vi "N4_201.vi"(4 "error in":T15, 7 "Command":T16) -> (0 "error out":T15, 3 "Response":T13)   [LabVIEW 2018]
uses:
  MOKO_LabViewLibrary/MokoLowLevel/MokoLowLovelControl/MLLC_Command.ctl
  MOKO_LabViewLibrary/MokoLowLevel/MokoLowLovelControl/MLLC_Error.ctl
  MOKO_LabViewLibrary/MokoLowLevel/MokoLowLovelControl/MLLC_Mode.ctl
  MOKO_LabViewLibrary/MokoLowLevel/MokoLowLovelControl/MLLC_Response.ctl
  MOKO_LabViewLibrary/MokoLowLevel/MokoLowLovelControl/MLLC_DriverName.ctl
  MOKO_LabViewLibrary/MokoLowLevel/MokoLowLovelControl/MLLC_Request.ctl
  MOKO_LabViewLibrary/MokoLowLevel/MokoLowLovelControl/MLLC_ErrorCode.ctl
  MOKO_LabViewLibrary/MokoLowLevel/MokoLowLovelControl/MLLC_ResponseInit.ctl
  MOKO_LabViewLibrary/MokoLowLevel/MokoLowLovelControl/MLLC_ConnectCluster.ctl
  MOKO_LabViewLibrary/MokoLowLevel/MokoLowLovelControl/MLLC_InterfaceType.ctl
  MOKO_LabViewLibrary/MokoLowLevel/MokoLowLovelControl/MLLC_OpenedSession.ctl
  MOKO_LabViewLibrary/MokoLowLevel/MokoLowLovelControl/MLLC_InterfaceSettings.ctl
  MOKO_LabViewLibrary/MokoLowLevel/MokoLowLovelControl/MLLC_InterfaceKind.ctl
  MOKO_LabViewLibrary/MokoLowLevel/MokoLowLovelControl/MLLC_Boolean.ctl
  MOKO_LabViewLibrary/MokoLowLevel/MokoLowLovelControl/MLLC_Delay.ctl
panel:
  in  "Settings":T8={"Connect"={"InterfaceType"=enum."VISA", "OpenedSession"="COM1", "InterfaceSettings"={"Interface"=enum."RS232", "EOS 4 read"=enum."LF (\\n)", "EOS 4 write"=enum."LF (\\n)", "TMO, ms"=10000, "Sett"=variant(cluster{"Baud Rate":u32, "Data Bits":u16, "Parity":u16, "Stop Bits":u16, "Flow Control":u16, "Eho":bool} {"Baud Rate"=75, "Data Bits"=0, "Parity"=0, "Stop Bits"=0, "Flow Control"=0, "Eho"=FALSE})}}, "SwitchOFF"=TRUE, "RangeAuto"=TRUE, "Range"=0.0}
  in  "ResponseInit":T9="N4-201"
  in  "Error Code":T10=5470
  in  "Request":T11="IDN?\n"
  in  "Driver Name":T12="N4_201"
  in  "Mode":T14=enum."Check"
  # "N4-201"
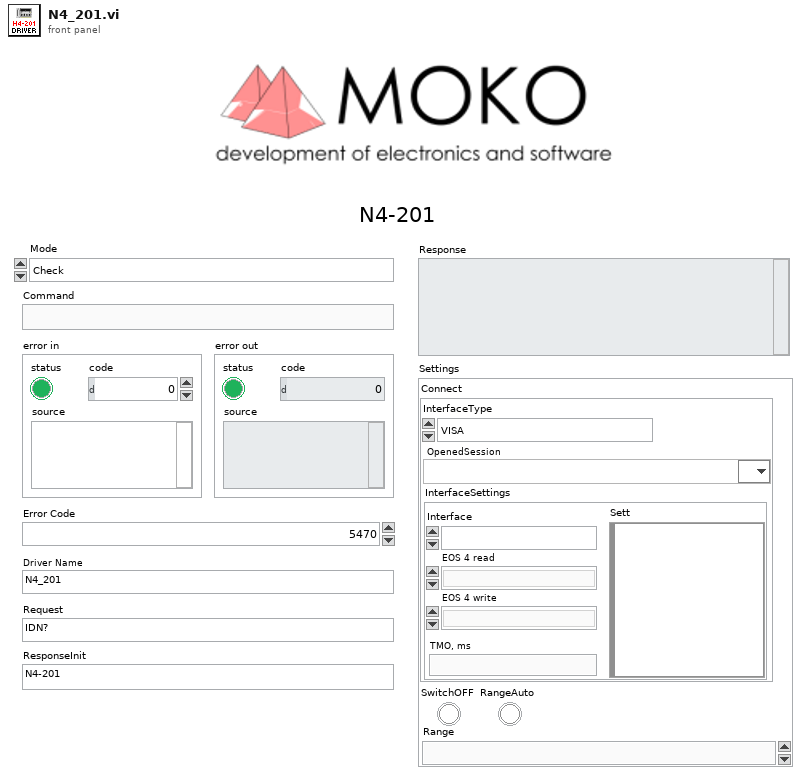
[diagram p1: front panel]
types:
  T1 = typedef "MLLC_ConnectCluster.ctl" = cluster{"InterfaceType":T2, "OpenedSession":T3, "InterfaceSettings":T4}
  T2 = typedef "MLLC_InterfaceType.ctl" = enum16{"VISA", "Prologix USB-GPIB"}
  T3 = typedef "MLLC_OpenedSession.ctl" = refnum<visa-resource-name>
  T4 = typedef "MLLC_InterfaceSettings.ctl" = cluster{"Interface":T5, "EOS 4 read":enum16{"Default (=EOS 4 write)", "CR (\\r)", "LF (\\n)", "None"}, "EOS 4 write":enum16{"CR+LF (\\r\\n)", "CR (\\r)", "LF (\\n)", "None"}, "TMO, ms":i32, "Sett":variant}
  T5 = typedef "MLLC_InterfaceKind.ctl" = enum16{"RS232", "GPIB", "USB", "Ethernet", "another"}
  T6 = typedef "MLLC_Boolean.ctl" = bool
  T7 = typedef "MLLC_Delay.ctl" = dbl
  T8 = cluster{"Connect":T1, "SwitchOFF":T6, "RangeAuto":T6, "Range":T7}
  T9 = typedef "MLLC_ResponseInit.ctl" = string
  T10 = typedef "MLLC_ErrorCode.ctl" = u32
  T11 = typedef "MLLC_Request.ctl" = string
  T12 = typedef "MLLC_DriverName.ctl" = string
  T13 = typedef "MLLC_Response.ctl" = string
  T14 = typedef "MLLC_Mode.ctl" = enum16{"get", "set", "close", "Init", "Check"}
  T15 = typedef "MLLC_Error.ctl" = errorcluster
  T16 = typedef "MLLC_Command.ctl" = string
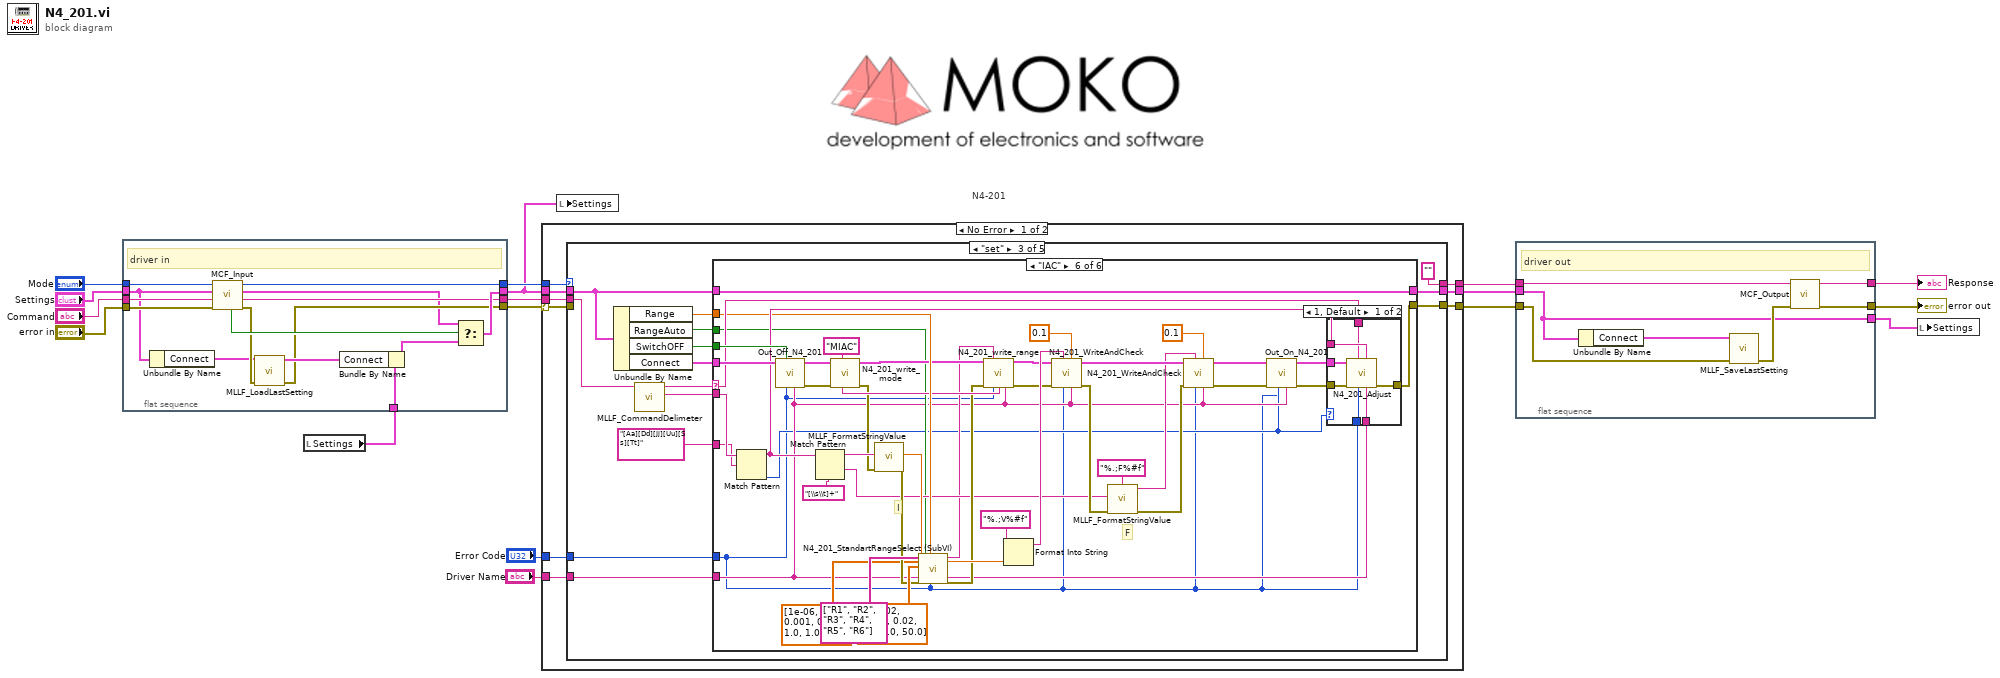
[diagram p0: block diagram]
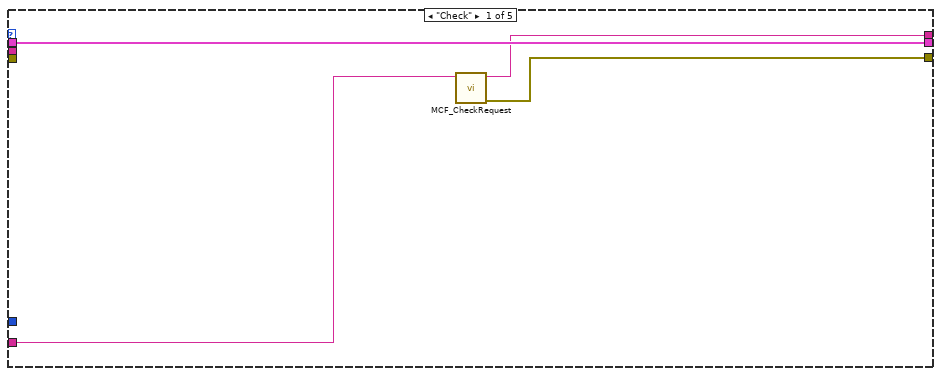
[diagram p2: hidden frame]
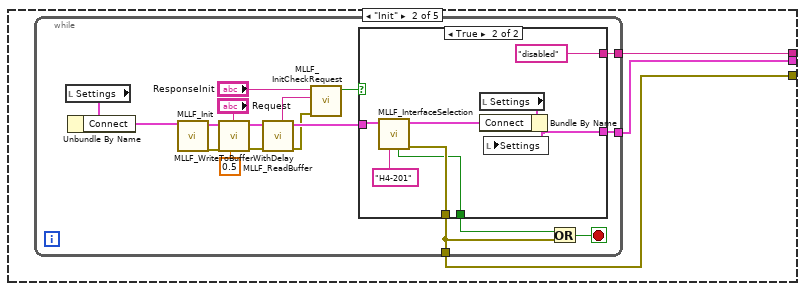
[diagram p3: hidden frame]
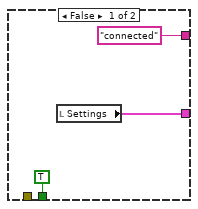
[diagram p4: hidden frame]
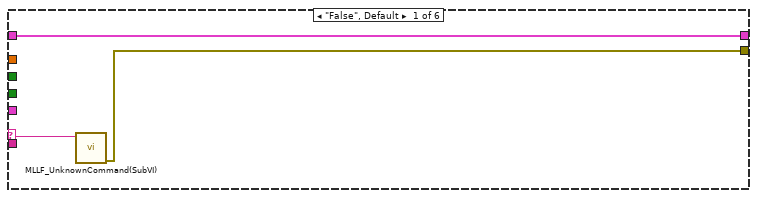
[diagram p5: hidden frame]
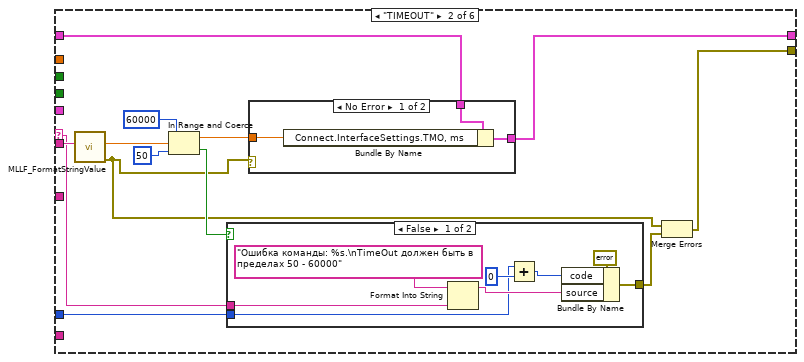
[diagram p6: hidden frame]
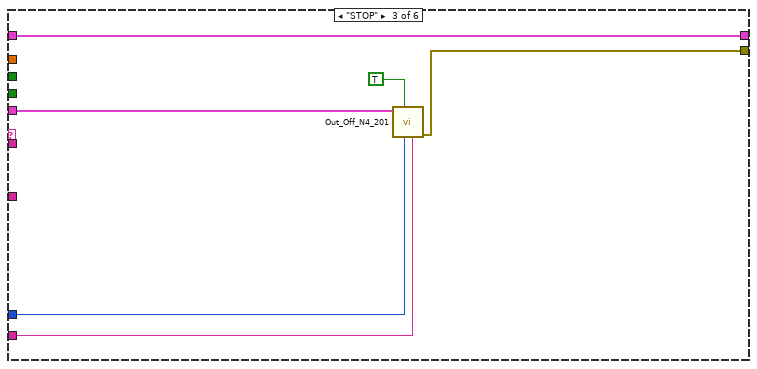
[diagram p9: hidden frame]
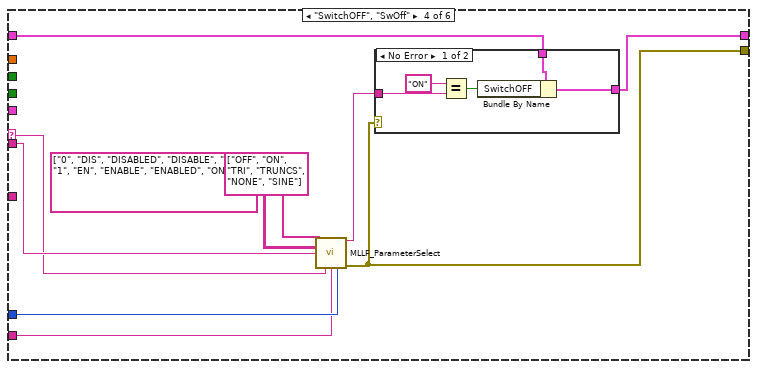
[diagram p10: hidden frame]
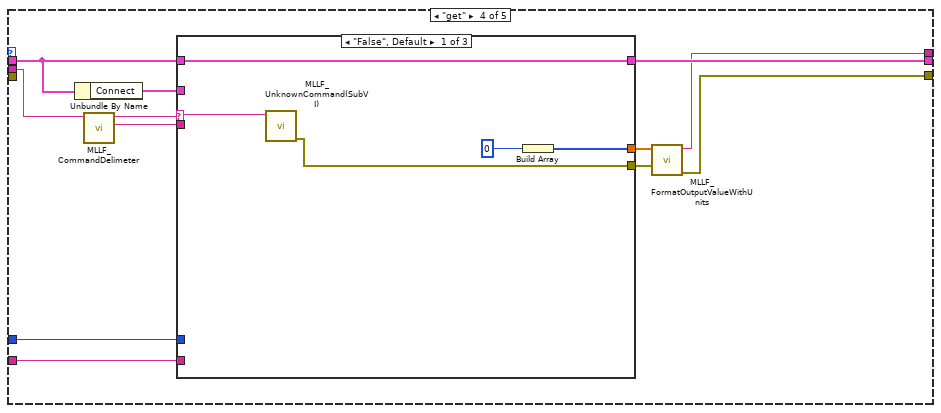
[diagram p14: hidden frame]
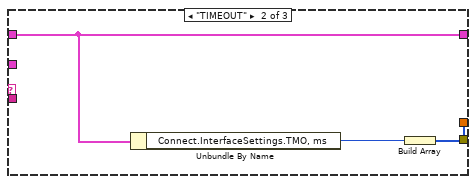
[diagram p15: hidden frame]
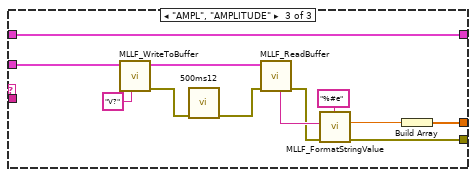
[diagram p16: hidden frame]
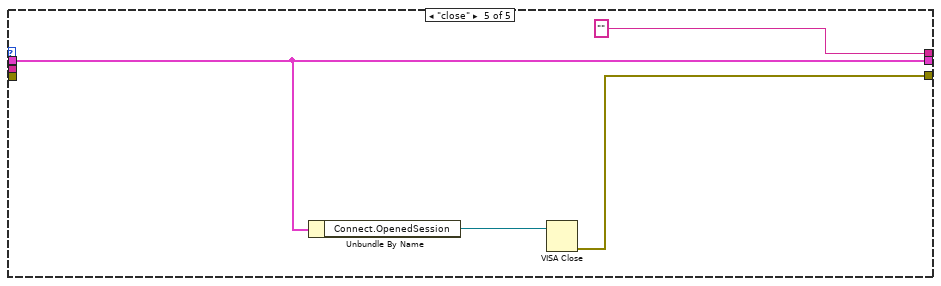
[diagram p17: hidden frame]
diagram:
  # "N4-201"
  n1 = flat-sequence {
    tunnel: [w24] -> w10
    tunnel: "Command" -> [w25]
    tunnel: "Mode" -> [w27]
    tunnel: "Settings" -> [w19]
    tunnel: [w29] -> w2
    tunnel: w1 -> [w28]
    tunnel: "error in" -> [w22]
    tunnel: [w21] -> w15
    tunnel: [w20] -> w9
    frame #0 {
      # "driver in"
      n2 = Unbundle By Name(w19) -> ("Connect"=w18:T1)
      n3 = call "MCF_Input.vi"("error in (no error)"=w22, "Command"=w25, "Mode"=w27) -> ("error out"=w23:errorcluster, "Command out"=w24:string, "Mode out"=w21:T14, "Boolean"=w26:bool)  [unwired: 5 in]
      n4 = call "MLLF_LoadLastSetting.vi"("Error In"=w23, "DriverConnectCluster in"=w18) -> ("Error Out"=w20:errorcluster, "DriverConnectCluster out"=w30:T1)  [unwired: 8 in]
      n5 = Bundle By Name(cluster=w28, "Connect"=w30) -> (w31:T8)
      n6 = Select(t=w19, s=w26, f=w31) -> (s? t:f=w29:T8)
    }
  }
  n7 = local read "Settings"() -> (w1:T8)
  n8 = case shown="No Error" w9 {
    selector: w9 -> [w36 w231]
    tunnel: [w38 w231] -> w6
    tunnel: w15 -> [w40 _]
    tunnel: [w39 _] -> w8
    tunnel: w10 -> [w37 _]
    tunnel: w2 -> [w33 w230]
    tunnel: "Error Code" -> [w35 _]
    tunnel: "Driver Name" -> [w34 _]
    tunnel: [w32 w230] -> w7
    frame No Error {
      n9 = case shown="\"set\"" w40 {
        tunnel: [w42 w47 "" ("String") w195 "" ("String")] -> w39
        tunnel: [w43 w45 w77 w194 w228] -> w38
        tunnel: w37 -> [_ _ w90 w205 _]
        tunnel: w36 -> [_ _ _ _ _]
        tunnel: w35 -> [_ _ w89 w202 _]
        tunnel: w34 -> [w41 _ w86 w201 _]
        tunnel: w33 -> [w44 _ w88 w204 w227]
        tunnel: [w44 w46 w87 w203 w227] -> w32
        frame "Check" {
          n10 = call "MCF_CheckRequest.vi"("Driver Name"=w41) -> ("Error Out"=w43:errorcluster, "Output String"=w42:string)  [unwired: 9 in]
        }
        frame "Init" {
          n11 = while {
            tunnel: [w58] -> w45
            tunnel: [w49] -> w46
            tunnel: [w48] -> w47
            stop <- w56 stop-if-true
            n12 = local read "Settings"() -> (w65:T8)
            n13 = Unbundle By Name(w65) -> ("Connect"=w59:T1)
            n14 = call "MLLF_Init.vi"("DriverConnect in"=w59) -> ("Error Out"=w61:errorcluster, "DriverConnect out"=w60:T1)  [unwired: 7 in]
            n15 = call "MLLF_WriteToBufferWithDelay.vi"("Delay Time ( 0,05 s)"=0.5 ("Delay Time (s)"), "Command"="Request", "Error In"=w61, "DriverConnect in"=w60) -> ("Error Out"=w54:errorcluster, "DriverConnect out"=w63:T1)  [unwired: 6 in]
            n16 = call "MLLF_ReadBuffer.vi"("Error In"=w54, "DriverConnect in"=w63) -> ("Error Out"=w51:errorcluster, "DriverConnect out"=w62:T1, "String"=w52:string)  [unwired: 6 in]
            n17 = call "MLLF_InitCheckRequest.vi"("error in (no error)"=w51, "Answer"=w52, "Response Init"="ResponseInit") -> ("Design"=w50:bool)  [unwired: 7 in, 1 out]
            n18 = case shown="True" w50 {
              tunnel: w62 -> [_ w75]
              tunnel: [_ w76] -> w58
              tunnel: [TRUE w69] -> w57
              tunnel: [w66 w71] -> w49
              tunnel: ["connected" "disabled"] -> w48
              frame False {
                n19 = local read "Settings"() -> (w66:T8)
              }
              frame True {
                n20 = call "MLLF_InterfaceSelection.vi"("Driver Name"="Н4-201" ("String"), "DriverConnect in"=w75) -> ("error out"=w76:T15, "DriverConnect out"=w73:T1, "stop init?"=w69:bool)  [unwired: 7 in]
                n21 = local read "Settings"() -> (w72:T8)
                n22 = Bundle By Name(cluster=w72, "Connect"=w73) -> (w71:T8)
                n23 = local write "Settings"(w71) -> ()
              }
            }
            n24 = Or(x=w57, y=w58) -> (x .or. y?=w56:bool)
          }
        }
        frame "set" {
          n25 = Unbundle By Name(w88) -> ("Range"=w80:T7, "RangeAuto"=w81:T6, "SwitchOFF"=w83:T6, "Connect"=w84:T1)
          n26 = call "MLLF_CommandDelimeter.vi"("command with param"=w90) -> ("param 1"=w78:string, "command"=w79:string)  [unwired: 7 in, 2 out]
          n27 = case shown="\"IAC\"" w79 {
            selector: w79 -> [w92 w94 _ w125 _ w164]
            tunnel: w78 -> [_ w97 _ w126 _ w168]
            tunnel: [w91 w100 w123 w129 _ w169] -> w77
            tunnel: w89 -> [_ w101 w121 w128 _ w142]
            tunnel: w88 -> [w93 w105 w124 w131 w141 w184]
            tunnel: [w93 w106 w124 w130 w141 w184] -> w87
            tunnel: w84 -> [_ _ w120 _ _ w185]
            tunnel: w86 -> [_ _ w122 w127 _ w144]
            tunnel: w83 -> [_ _ _ _ _ w175]
            tunnel: "[Aa][Dd][Jj][Uu][Ss][Tt]" ("regular expression") -> [_ _ _ _ _ w163]
            tunnel: w81 -> [_ _ _ _ _ w151]
            tunnel: w80 -> [_ _ _ _ _ w162]
            frame "False", Default {
              n28 = call "MLLF_UnknownCommand(SubVI).vi"("Unknown command"=w92) -> ("error out"=w91:errorcluster)  [unwired: 10 in]
            }
            frame "TIMEOUT" {
              n29 = call "MLLF_FormatStringValue.vi"("String Value"=w97) -> ("error out"=w95:T15, "number"=w96:dbl)  [unwired: 8 in, 1 out]
              n30 = In Range and Coerce(upper limit=60000, x=w96, lower limit=50) -> (coerced(x)=w102:dbl, In Range?=w98:bool)
              n31 = case shown="False" w98 {
                tunnel: [w113 _] -> w99
                tunnel: w101 -> [w112 _]
                tunnel: w94 -> [w111 _]
                frame False {
                  n32 = Format Into String(format string="Ошибка команды: %s.\nTimeOut должен быть в пределах 50 - 60000", w111) -> (resulting string=w115:string)  [unwired: 2 in, 1 out]
                  n33 = Add(x=w112, y=0) -> (x+y=w116:T10)
                  n34 = Bundle By Name(cluster=errorcluster {"status"=TRUE, "code"=0, "source"=""} ("error out"), "code"=w116, "source"=w115) -> (w113:errorcluster)
                }
                frame True {
                }
              }
              n35 = case shown="No Error" w95 {
                tunnel: [w109 w110] -> w106
                tunnel: w105 -> [w108 w110]
                tunnel: w102 -> [w107 _]
                frame No Error {
                  n36 = Bundle By Name(cluster=w108, "Connect.InterfaceSettings.TMO, ms"=w107) -> (w109:T8)
                }
                frame Error {
                }
              }
              n37 = Merge Errors(w95, w99) -> (w100:errorcluster)
            }
            frame "STOP" {
              n38 = call "Out_Off_N4_201.vi"("Driver Name"=w122, "Error Code"=w121, "SwitchOFF"=TRUE, "DriverConnect in"=w120) -> ("error out"=w123:T15)  [unwired: 6 in, 1 out]
            }
            frame "SwitchOFF", "SwOff" {
              n39 = call "MLLF_ParameterSelect.vi"("Command to equipment"=string[] ["OFF", "ON", "TRI", "TRUNCS", "NONE", "SINE"] ("Parameters"), "Names"=string[][] [["0", "DIS", "DISABLED", "DISABLE", "OFF"], ["1", "EN", "ENABLE", "ENABLED", "ON"]], "Input"=w126, "Command"=w125, "Driver Name"=w127, "Error Code"=w128) -> ("Choice"=w134:string, "Error Out"=w129:errorcluster)  [unwired: 8 in]
              n40 = case shown="No Error" w129 {
                tunnel: w134 -> [w139 _]
                tunnel: w131 -> [w137 w140]
                tunnel: [w136 w140] -> w130
                frame No Error {
                  n41 = Equal?(x="ON", y=w139) -> (x = y?=w135:bool)
                  n42 = Bundle By Name(cluster=w137, "SwitchOFF"=w135) -> (w136:T8)
                }
                frame Error {
                }
              }
            }
            frame "<----MAIN FUNCTIONS---->" {
            }
            frame "IAC" {
              w157 = "MIAC" ("String")
              # "F"
              # "I"
              n43 = Match Pattern(string=w168, regular expression=w163) -> (before substring=w165:string, offset past match=w143:i32)  [unwired: 1 in, 2 out]
              n44 = call "Out_Off_N4_201.vi"("Driver Name"=w144, "Error Code"=w142, "SwitchOFF"=w175, "DriverConnect in"=w185) -> ("error out"=w156:T15, "DriverConnect out"=w158:T1)  [unwired: 6 in]
              n45 = Match Pattern(string=w165, regular expression="[\\s\\t]+") -> (before substring=w182:string, after substring=w153:string)  [unwired: 1 in, 2 out]
              n46 = call "N4_201_write_mode.vi"("Command"=w157, "error in"=w156, "DriverConnect in"=w158) -> ("error out"=w155:T15, "DriverConnect out"=w161:T1)  [unwired: 6 in, 1 out]
              n47 = call "MLLF_FormatStringValue.vi"("error in"=w155, "String Value"=w182) -> ("error out"=w178:T15, "number"=w177:dbl)  [unwired: 7 in, 1 out]
              n48 = call "N4_201_StandartRangeSelect (SubVI).vi"("RangeCommand"=string[] ["R1", "R2", "R3", "R4", "R5", "R6"], "ScaleArray"=dbl[] [1e-06, 0.001, 0.001, 0.001, 1.0, 1.0], "RangeDigit"=dbl[] [0.0002, 0.002, 0.02, 0.2, 2.0, 50.0], "Control Point"=w177, "error in"=w178, "RangeAuto"=w151, "Range"=w162, "Error Code"=w142, "Driver Name"=w144) -> ("R/O"=w152:string, "ScaledValue"=w170:dbl, "error out"=w154:errorcluster)  [unwired: 8 in]
              n49 = call "N4_201_write_range.vi"("DriverConnect in"=w161, "Command range"=w152, "error in"=w154, "Error Code"=w142, "Command mode"=w157, "Driver Name"=w144) -> ("DriverConnect out"=w160:T1, "error out"=w159:T15)  [unwired: 7 in, 1 out]
              n50 = Format Into String(format string="%.;V%#f", w170) -> (resulting string=w174:string)  [unwired: 2 in, 1 out]
              n51 = call "N4_201_WriteAndCheck.vi"("Driver Name"=w144, "Command Time (s)"=0.1, "Error Code"=w142, "Command"=w174, "error in"=w159, "DriverConnect in"=w160) -> ("error out"=w167:T15, "DriverConnect out"=w173:T1)  [unwired: 4 in]
              n52 = call "MLLF_FormatStringValue.vi"("error in"=w167, "String Value"=w153, "Format"="%.;F%#f" ("format string")) -> ("error out"=w166:T15, "String Value Formated"=w172:T16)  [unwired: 6 in, 1 out]
              n53 = call "N4_201_WriteAndCheck.vi"("Driver Name"=w144, "Command Time (s)"=0.1, "Error Code"=w142, "Command"=w172, "error in"=w166, "DriverConnect in"=w173) -> ("error out"=w147:T15, "DriverConnect out"=w148:T1)  [unwired: 4 in]
              n54 = call "Out_On_N4_201.vi"("Driver Name"=w144, "Error Code"=w142, "ADJUST"=w143, "error in"=w147, "DriverConnect in"=w148) -> ("error out"=w145:T15, "DriverConnect out"=w146:T1)  [unwired: 5 in]
              n55 = case shown="1, Default" w143 {
                tunnel: [w192 w193] -> w169
                tunnel: w142 -> [w191 _]
                tunnel: w144 -> [w190 _]
                tunnel: w165 -> [w189 _]
                tunnel: w164 -> [w188 _]
                tunnel: w146 -> [w187 _]
                tunnel: w145 -> [w186 w193]
                frame 1, Default {
                  n56 = call "N4_201_Adjust.vi"("Driver Name"=w190, "ValueIn"=w189, "Error Code"=w191, "Command"=w188, "error in"=w186, "DriverConnect in"=w187) -> ("error out"=w192:T15)  [unwired: 4 in, 1 out]
                }
                frame -1 {
                }
              }
            }
          }
        }
        frame "get" {
          n57 = Unbundle By Name(w204) -> ("Connect"=w198:T1)
          n58 = call "MLLF_CommandDelimeter.vi"("command with param"=w205) -> ("param 1"=w196:string, "command"=w197:string)  [unwired: 7 in, 2 out]
          n59 = case shown="\"False\", Default" w197 {
            selector: w197 -> [w207 _ _]
            tunnel: w196 -> [_ _ _]
            tunnel: [w206 _ w214] -> w200
            tunnel: w202 -> [_ _ _]
            tunnel: [w210 w213 w225] -> w203
            tunnel: w204 -> [w210 w213 w225]
            tunnel: [w208 w211 w224] -> w199
            tunnel: w198 -> [_ _ w217]
            tunnel: w201 -> [_ _ _]
            frame "False", Default {
              n60 = call "MLLF_UnknownCommand(SubVI).vi"("Unknown command"=w207) -> ("error out"=w206:errorcluster)  [unwired: 10 in]
              n61 = Build Array(0 ("TimeOut")) -> (w208:i32[])
            }
            frame "TIMEOUT" {
              n62 = Unbundle By Name(w213) -> ("Connect.InterfaceSettings.TMO, ms"=w212:i32)
              n63 = Build Array(w212) -> (w211:i32[])
            }
            frame "AMPL", "AMPLITUDE" {
              n64 = call "MLLF_WriteToBuffer.vi"("String"="V?" ("Error Query"), "DriverConnect in"=w217) -> ("error out"=w222:T15, "DriverConnect out"=w218:T1)  [unwired: 6 in]
              n65 = call "500ms12"("error in (no error)"=w222) -> ("error out"=w223:errorcluster)  [unwired: 10 in]
              n66 = call "MLLF_ReadBuffer.vi"("Error In"=w223, "DriverConnect in"=w218) -> ("Error Out"=w215:errorcluster, "String"=w220:string)  [unwired: 6 in, 1 out]
              n67 = call "MLLF_FormatStringValue.vi"("error in"=w215, "String Value"=w220, "Format"="%#e" ("format string")) -> ("error out"=w214:T15, "number"=w216:dbl)  [unwired: 6 in, 1 out]
              n68 = Build Array(w216) -> (w224:dbl[])
            }
          }
          n69 = call "MLLF_FormatOutputValueWithUnits.vi"("error in"=w200, "ValuesIn"=w199) -> ("error out"=w194:T15, "Result string"=w195:T16)  [unwired: 8 in]
        }
        frame "close" {
          n70 = Unbundle By Name(w227) -> ("Connect.OpenedSession"=w229:T3)
          n71 = VISA Close(VISA resource name=w229) -> (error out=w228:errorcluster)  [unwired: 1 in]
        }
      }
    }
    frame Error {
    }
  }
  n72 = local write "Settings"(w2) -> ()
  n73 = flat-sequence {
    tunnel: [w238] -> w5
    tunnel: w8 -> [w237]
    tunnel: w6 -> [w232]
    tunnel: w7 -> [w233]
    tunnel: [w233] -> w3
    tunnel: [w234] -> w4
    frame #0 {
      # "driver out"
      n74 = Unbundle By Name(w233) -> ("Connect"=w236:T1)
      n75 = call "MLLF_SaveLastSetting.vi"("error in"=w232, "DriverConnectCluster in"=w236) -> ("error out"=w235:T15)  [unwired: 8 in, 1 out]
      n76 = call "MCF_Output.vi"("Error In"=w235, "Input"=w237) -> ("Error Out"=w234:errorcluster, "Output"=w238:string)  [unwired: 8 in]
    }
  }
  n77 = local write "Settings"(w3) -> ()
  "error out" <- w4
  "Response" <- w5
